vi "Merge LV and PCAP network info.vi"(8 "error in (no error)":errorcluster, 10 "pcap information":T2[](array[typedef]), 11 "Network information":T1[](array[typedef])) -> (0 "error out":errorcluster, 2 "Selection string":string[](array[string]), 3 "Merged":T1[](array[typedef]))   [LabVIEW 2020]
uses:
  TypeDef/pcap device details.ctl
  TypeDef/Network adaptor details.ctl
panel:
  out "Boolean":bool
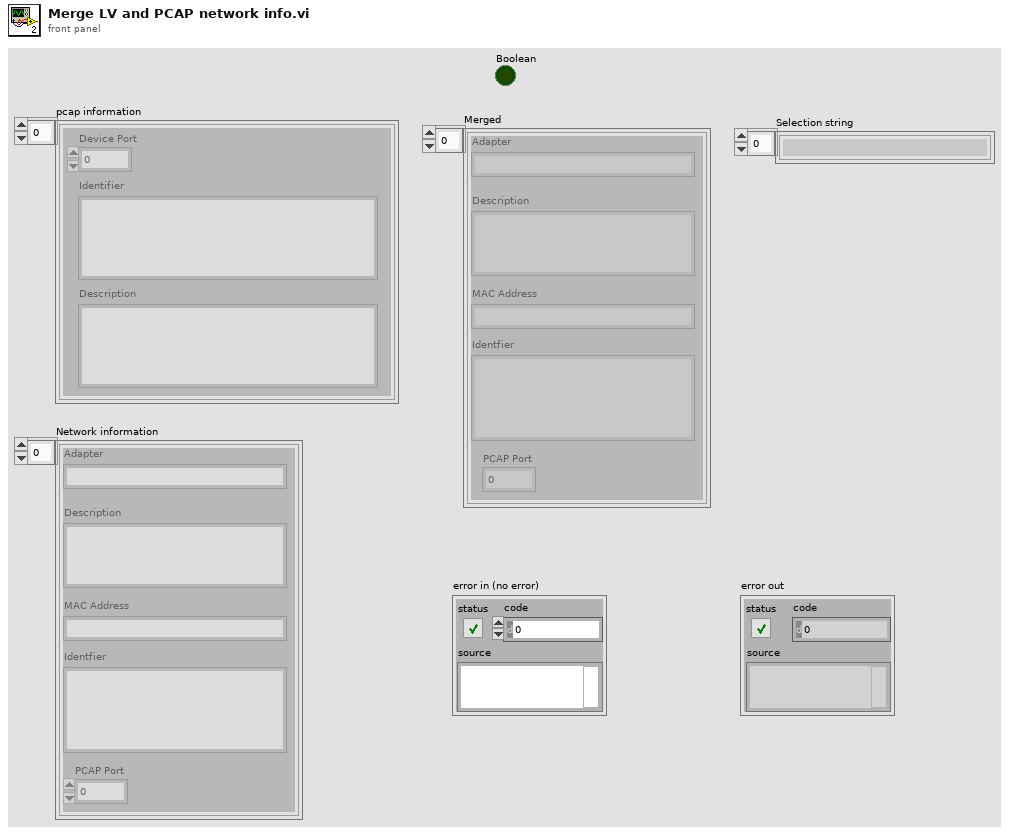
[diagram p1: front panel]
types:
  T1 = typedef "Network adaptor details.ctl" = cluster{"Adapter":string, "Description":string, "MAC Address":string, "Identfier":string, "PCAP Port":u32}
  T2 = typedef "pcap device details.ctl" = cluster{"Device Port":u32, "Identifier":string, "Description":string}
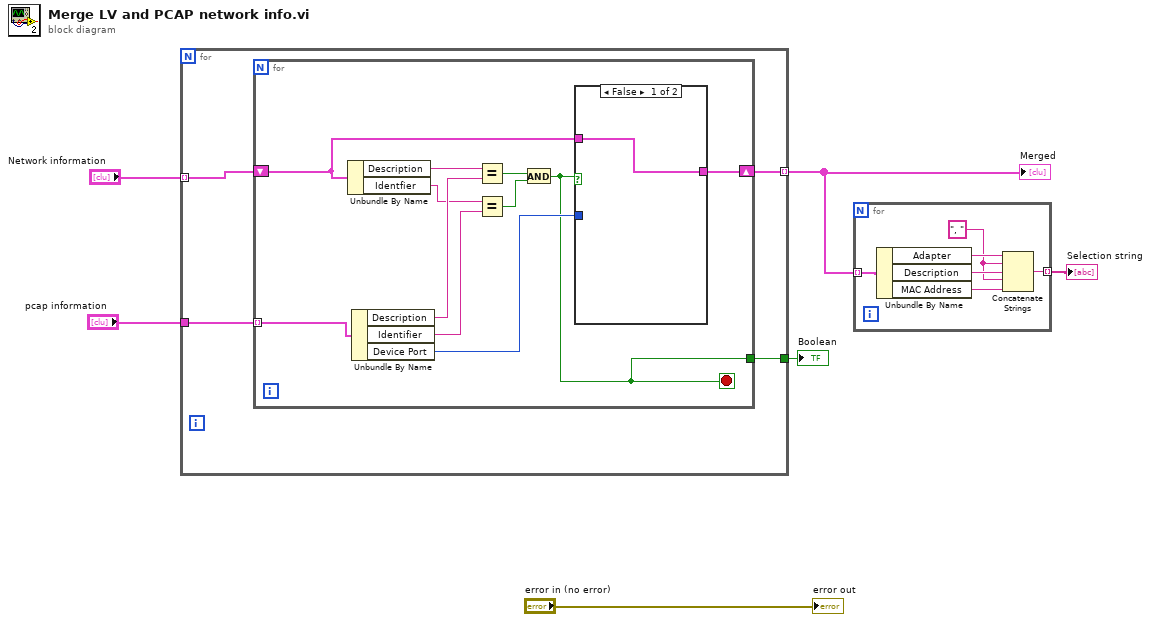
[diagram p0: block diagram]
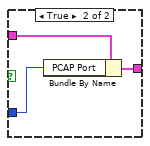
[diagram p2: hidden frame]
diagram:
  n1 = for {
    tunnel: "pcap information" -> [w8]
    tunnel: "Network information" -> [w10] mode=indexing
    tunnel: [w9] -> w4 mode=indexing
    tunnel: [w7] -> w1
    n2 = for {
      tunnel: w8 -> [w12] mode=indexing
      shift-right: [w13] -> w9
      shift-left: w10 -> [w15]
      tunnel: [w11] -> w7
      stop <- w11 stop-if-true
      n3 = Unbundle By Name(w15) -> ("Description"=w21:string, "Identfier"=w19:string)
      n4 = Unbundle By Name(w12) -> ("Description"=w20:string, "Identifier"=w18:string, "Device Port"=w14:u32)
      n5 = Equal?(x=w21, y=w20) -> (x = y?=w17:bool)
      n6 = Equal?(x=w19, y=w18) -> (x = y?=w16:bool)
      n7 = And(x=w17, y=w16) -> (x .and. y?=w11:bool)
      n8 = case shown="False" w11 {
        tunnel: w15 -> [w22 w25]
        tunnel: w14 -> [_ w24]
        tunnel: [w22 w23] -> w13
        frame False {
        }
        frame True {
          n9 = Bundle By Name(cluster=w25, "PCAP Port"=w24) -> (w23:T1)
        }
      }
    }
  }
  "Merged" <- w4
  "Boolean" <- w1
  n10 = for {
    tunnel: w4 -> [w31] mode=indexing
    tunnel: [w26] -> w3 mode=indexing
    w27 = ", " ("string")
    n11 = Unbundle By Name(w31) -> ("Adapter"=w30:string, "Description"=w29:string, "MAC Address"=w28:string)
    n12 = Concatenate Strings(w30, w27, w29, w27, w28) -> (w26:string)
  }
  "Selection string" <- w3
  "error out" <- "error in (no error)"
